vi "Connect_disconnect.vi"(1 "PXI_Trig0 of ao1":tag="/6733_1/PXI_Trig0", 2 "Connect?":bool, 3 "Fast AO lines":i32=2) -> (0 "error out":errorcluster)   [LabVIEW 2018]
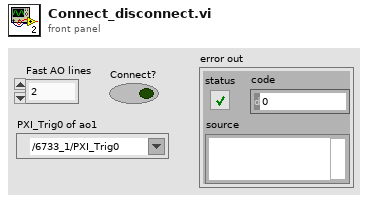
[diagram p1: front panel]
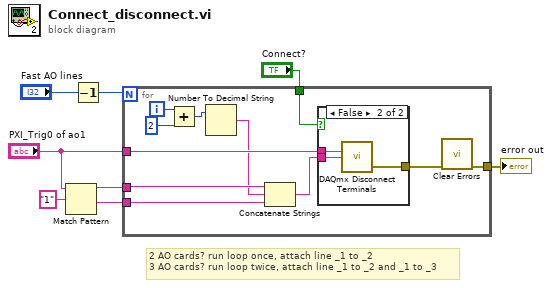
[diagram p0: block diagram]
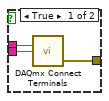
[diagram p2: hidden frame]
diagram:
  # "2 AO cards? run loop once, attach line _1 to _2\n3 AO cards? run loop twice, attach line _1 to _2 and _1 to _3"
  n1 = Match Pattern(string="PXI_Trig0 of ao1", regular expression="1") -> (before substring=w7:string, after substring=w3:string)  [unwired: 1 in, 2 out]
  n2 = Decrement(x="Fast AO lines") -> (x-1=w2:i32)
  n3 = for {
    N: w2 -> [_]
    tunnel: "PXI_Trig0 of ao1" -> [w18]
    tunnel: w7 -> [w17]
    tunnel: [w11] -> w8
    tunnel: "Connect?" -> [w10]
    tunnel: w3 -> [w9]
    i -> [w16]
    n4 = Add(x=w16, y=2) -> (x+y=w14:i32)
    n5 = Number To Decimal String(number=w14) -> (decimal integer string=w13:string)  [unwired: 1 in]
    n6 = Concatenate Strings(w17, w13, w9) -> (w12:string)
    n7 = case shown="False" w10 {
      tunnel: [w22 w25] -> w19
      tunnel: w18 -> [w21 w24]
      tunnel: w12 -> [w20 w23]
      frame True {
        n8 = call <vilib>:"DAQmx Connect Terminals.vi"("source terminal"=w21, "destination terminal"=w20) -> ("error out"=w22:errorcluster)  [unwired: 13 in]
      }
      frame False {
        n9 = call <vilib>:"DAQmx Disconnect Terminals.vi"("source terminal"=w24, "destination terminal"=w23) -> ("error out"=w25:errorcluster)  [unwired: 13 in]
      }
    }
    n10 = call <vilib>:"Clear Errors.vi"("error in (no error)"=w19) -> ("error out"=w11:errorcluster)  [unwired: 5 in, 1 out]
  }
  "error out" <- w8
